vi "Delete File.vi"(0 "Path":path, 11 "error in (no error)":errorcluster) -> (15 "error out":errorcluster)   [LabVIEW 2021, in "Path Functions.lvlib"]
uses:
  Path Functions.lvlib
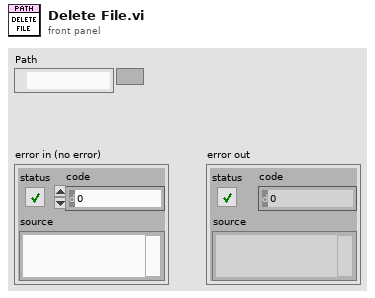
[diagram p1: front panel]
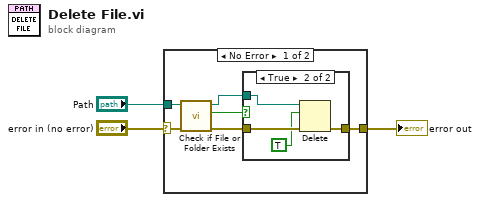
[diagram p0: block diagram]
diagram:
  n1 = case shown="No Error" "error in (no error)" {
    selector: "error in (no error)" -> [w6 w15]
    tunnel: "Path" -> [w9 _]
    tunnel: [w4 w15] -> w1
    frame No Error {
      n2 = call <vilib>:"Check if File or Folder Exists.vi"("error in (no error)"=w6, "path"=w9) -> ("error out"=w5:errorcluster, "file or folder exists?"=w7:bool, "dup path"=w8:path)  [unwired: 7 in]
      n3 = case shown="True" w7 {
        tunnel: w8 -> [_ w14]
        tunnel: w5 -> [w10 w13]
        tunnel: [w10 w12] -> w4
        frame False {
        }
        frame True {
          n4 = Delete(path (use dialog)=w14, entire hierarchy (F)=TRUE, error in=w13) -> (error out=w12:errorcluster)  [unwired: 2 in, 2 out]
        }
      }
    }
    frame Error {
    }
  }
  "error out" <- w1
